vi "LoadINIFile.vi"(8 "error in":errorcluster, 11 "Sequence Context In":refnum<k7>) -> (0 "error out":errorcluster)   [LabVIEW 2019]
uses:
  <vilib>/Utility/config.llb/NI_LVConfig.lvlib
  <vilib>/addons/TestStand/_TSUtility.llb/TestStand - Set Property Value (String).vi
  <vilib>/addons/TestStand/_TSUtility.llb/TestStand - Set Property Value (Number).vi
  <vilib>/Utility/config.llb/Read Key (String).vi
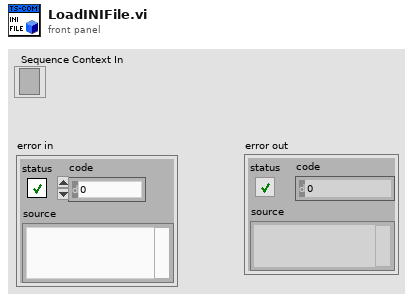
[diagram p1: front panel]
types:
  T1 = typedef "NI_LVConfig.lvlib/Config Data RefNum.ctl" = refnum<k1>
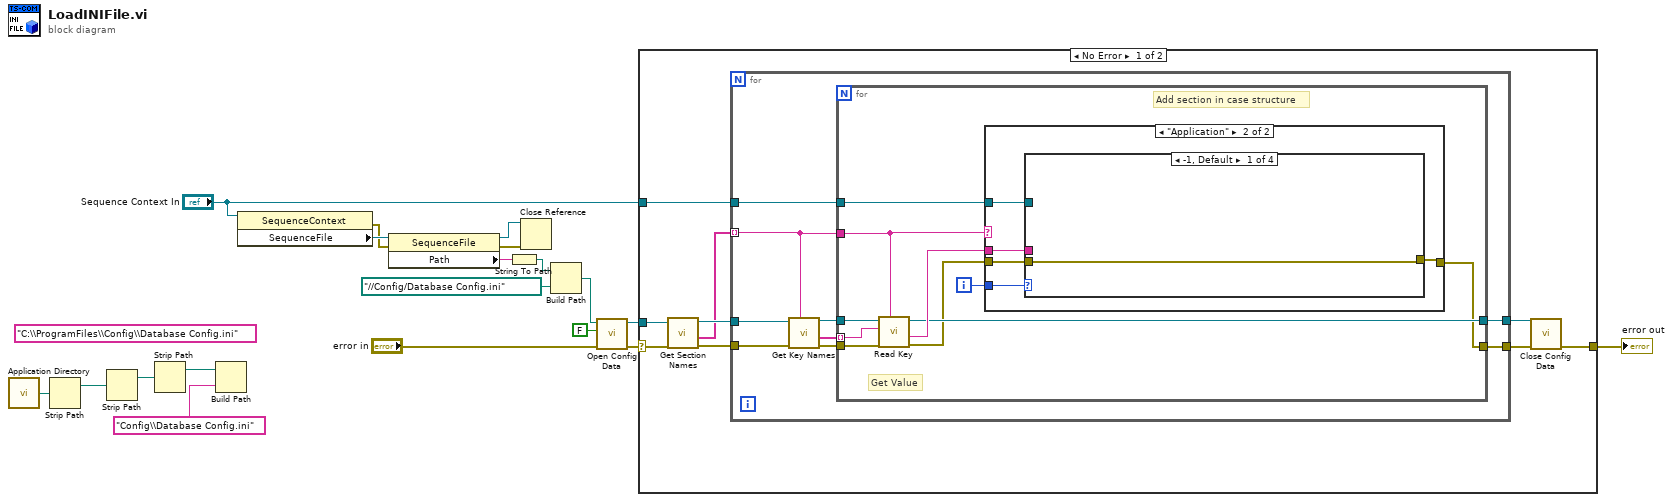
[diagram p0: block diagram]
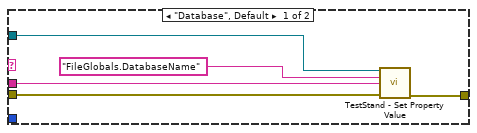
[diagram p2: hidden frame]
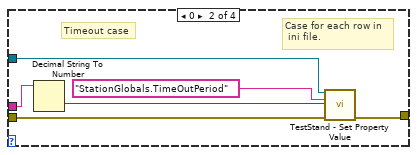
[diagram p3: hidden frame]
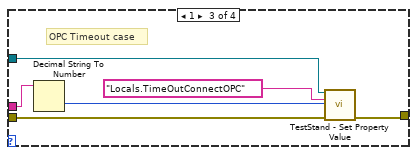
[diagram p4: hidden frame]
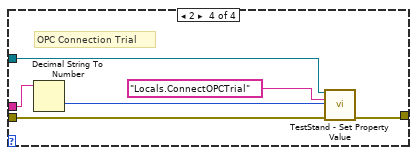
[diagram p5: hidden frame]
diagram:
  (unwired) "C:\\ProgramFiles\\Config\\Database Config.ini"
  n1 = call <vilib>:"Application Directory.vi"() -> ("Application Directory"=w19:path)
  n2 = Strip Path(path=w19) -> (stripped path=w18:path)  [unwired: 1 out]
  n3 = Strip Path(path=w18) -> (stripped path=w11:path)  [unwired: 1 out]
  n4 = Strip Path(path=w11) -> (stripped path=w10:path)  [unwired: 1 out]
  n5 = Build Path(base path=w10, name or relative path="Config\\Database Config.ini") -> ()  [unwired: 1 out]
  n6 = property class="SequenceContext"(reference="Sequence Context In") -> (error out=w7:errorcluster, "SequenceFile"=w8:refnum<k7>)  [unwired: 1 in, 1 out]
  n7 = property class="SequenceFile"(reference=w8, error in=w7) -> (reference out=w1:refnum<k7>, error out=w2:errorcluster, "Path"=w6:string)
  n8 = String To Path(string=w6) -> (path=w5:path)
  n9 = Close Reference(reference=w1, error in (no error)=w2) -> ()  [unwired: 1 out]
  n10 = Build Path(base path=w5, name or relative path=path "../../Config/Database Config.ini") -> (appended path=w3:path)
  n11 = call <vilib>:"Open Config Data.vi"("error in (no error)"="error in", "create file if necessary (T)"=FALSE, "configuration file path"=w3) -> ("error out"=w13:errorcluster, "refnum"=w14:T1)  [unwired: 6 in, 1 out]
  n12 = case shown="No Error" w13 {
    selector: w13 -> [w25 w77]
    tunnel: w14 -> [w28 _]
    tunnel: "Sequence Context In" -> [w21 _]
    tunnel: [w20 w77] -> w12
    frame No Error {
      n13 = call <vilib>:"Get Section Names.vi"("error in (no error)"=w25, "refnum"=w28) -> ("error out"=w27:errorcluster, "section names"=w24:string[], "refnum out"=w26:T1)  [unwired: 7 in]
      n14 = for {
        tunnel: w27 -> [w37]
        tunnel: w26 -> [w36]
        tunnel: w24 -> [w32] mode=indexing
        tunnel: [w31] -> w23
        tunnel: [w30] -> w22
        tunnel: w21 -> [w29]
        n15 = call <vilib>:"Get Key Names.vi"("section"=w32, "error in (no error)"=w37, "refnum"=w36) -> ("error out"=w34:errorcluster, "key names"=w35:string[], "refnum out"=w33:T1)  [unwired: 5 in, 1 out]
        n16 = for {
          tunnel: w35 -> [w46] mode=indexing
          tunnel: w34 -> [w47]
          tunnel: w33 -> [w45]
          tunnel: w32 -> [w44]
          tunnel: [w39] -> w31
          tunnel: [w42] -> w30
          tunnel: w29 -> [w41]
          i -> [w38]
          # "Add section in case structure"
          # "Get Value"
          n17 = call-poly <vilib>:"Read Key.vi"("section"=w44, "error in (no error)"=w47, "key"=w46, "refnum"=w45) -> ("error out"=w40:errorcluster, "value"=w43:string, "refnum out"=w42:T1)  [unwired: 4 in, 1 out]
          n18 = case shown="\"Application\"" w44 {
            tunnel: w43 -> [w52 w55]
            tunnel: w41 -> [w48 w56]
            tunnel: w40 -> [w51 w57]
            tunnel: [w49 w53] -> w39
            tunnel: w38 -> [_ w54]
            frame "Database", Default {
              n19 = call-poly <vilib>:"TestStand - Set Property Value.vi"("Sequence Context In"=w48, "Lookup String"="FileGlobals.DatabaseName", "New Value"=w52, "error in (no error)"=w51) -> ("error out"=w49:errorcluster)  [unwired: 10 in, 1 out]
            }
            frame "Application" {
              n20 = case shown="-1, Default" w54 {
                tunnel: w57 -> [w58 w64 w70 w76]
                tunnel: w56 -> [_ w62 w68 w74]
                tunnel: w55 -> [_ w61 w67 w73]
                tunnel: [w58 w59 w65 w71] -> w53
                frame -1, Default {
                }
                frame 0 {
                  # "Timeout case"
                  # "Case for each row in\n ini file."
                  n21 = Decimal String To Number(string=w61) -> (number=w60:i32)  [unwired: 2 in, 1 out]
                  n22 = call-poly <vilib>:"TestStand - Set Property Value.vi"("Sequence Context In"=w62, "Lookup String"="StationGlobals.TimeOutPeriod", "New Value"=w60, "error in (no error)"=w64) -> ("error out"=w59:errorcluster)  [unwired: 10 in, 1 out]
                }
                frame 1 {
                  # "OPC Timeout case"
                  n23 = Decimal String To Number(string=w67) -> (number=w66:i32)  [unwired: 2 in, 1 out]
                  n24 = call-poly <vilib>:"TestStand - Set Property Value.vi"("Sequence Context In"=w68, "Lookup String"="Locals.TimeOutConnectOPC", "New Value"=w66, "error in (no error)"=w70) -> ("error out"=w65:errorcluster)  [unwired: 10 in, 1 out]
                }
                frame 2 {
                  # "OPC Connection Trial"
                  n25 = Decimal String To Number(string=w73) -> (number=w72:i32)  [unwired: 2 in, 1 out]
                  n26 = call-poly <vilib>:"TestStand - Set Property Value.vi"("Sequence Context In"=w74, "Lookup String"="Locals.ConnectOPCTrial", "New Value"=w72, "error in (no error)"=w76) -> ("error out"=w71:errorcluster)  [unwired: 10 in, 1 out]
                }
              }
            }
          }
        }
      }
      n27 = call <vilib>:"Close Config Data.vi"("error in (no error)"=w23, "refnum"=w22) -> ("error out"=w20:errorcluster)  [unwired: 8 in, 1 out]
    }
    frame Error {
    }
  }
  "error out" <- w12
